vi "Global Variable.vi"() -> ()   [LabVIEW 2018]
panel:
  out "PicoScope Device Info":T1
  out "BLE Data":string
  out "PicoScope Correction":i32
  out "FTDI RS232 Handle  RFID":u32
  out "Baccode MEM":string
  in  "VI Refnum Main":refnum<vi>
  out "Steps Cnt":u16
  out "Sequencer Path":path[](array[path])=[path "***", path "***", path "***", path "***", path "***", path "***", path "***", path "***", path "***", path "***"]
  out "logFile Path":refnum<file>
  out "Reset BARCODE":bool
  out "Retest Nmb":i16
  out "Boards False":u32
  out "Boards Pass":u32
  out "Boards Total":u32
  out "DB Dir Path":path caption="Sequenser INI Config File Path"
  out "Config":string="***"
  out "Board":string="***"
  out "Customer":string="***"
  out "Gen Err Cnt":u16
  out "Cancel by operator":bool
  out "RFID Power":u16
  out "Retest Step Nmb":u32
  out "Retest ON":bool
  out "Retest Cnt":i16
  out "Rd PID RFID":string
  out "COM Port RFID":refnum<visa-resource-name>
  in  "VI Ref PicoScope Read":refnum<vi>
  out "Test Gen Status":bool
  out "COM Port BLE":refnum<visa-resource-name>
  out "Rd PID Ble":string
  out "ADC Offset":i32
  out "Test Time":u32
  out "Test Stop Time":u32
  out "Test Start Time":u32
  out "Array_Measurement":dbl[](array[numeric]) format="%#.3g"
  out "Rd PID":string
  out "Wr PID":string
  out "COM Port FTDI RS232":refnum<visa-resource-name>
  out "PowSupply ON/OFF":bool
  out "GPIO Mode LUT":bool[](array[boolean])
  out "PicoScope Max Adc Value":i16
  out "PicoScope Handle":u32
  in  "Step Test Result":enum16{"Idle", "PASS", "FALSE"}(ring)
  out "Report Active Lines Cnt":u32
  out "Report Step Nmb":u32
  out "Active Lines Cnt":u32
  out "VISA Resource Name BK-5492C":string
  out "VISA Resource Name BK-9202":string
  out "Simbol Array":u32[](array[numeric])
  out "Current Step Nmb":u32
  out "Steps Nmb":u32
  out "FTDI RS232 Handle":u32
  out "FTDI SPI Handle":u32
  out "Array Errors":errorcluster[](array[cluster])
  out "Sys ERR":bool
  out "Dev List":string[](array[string])
  out "System Status":T2(ring)
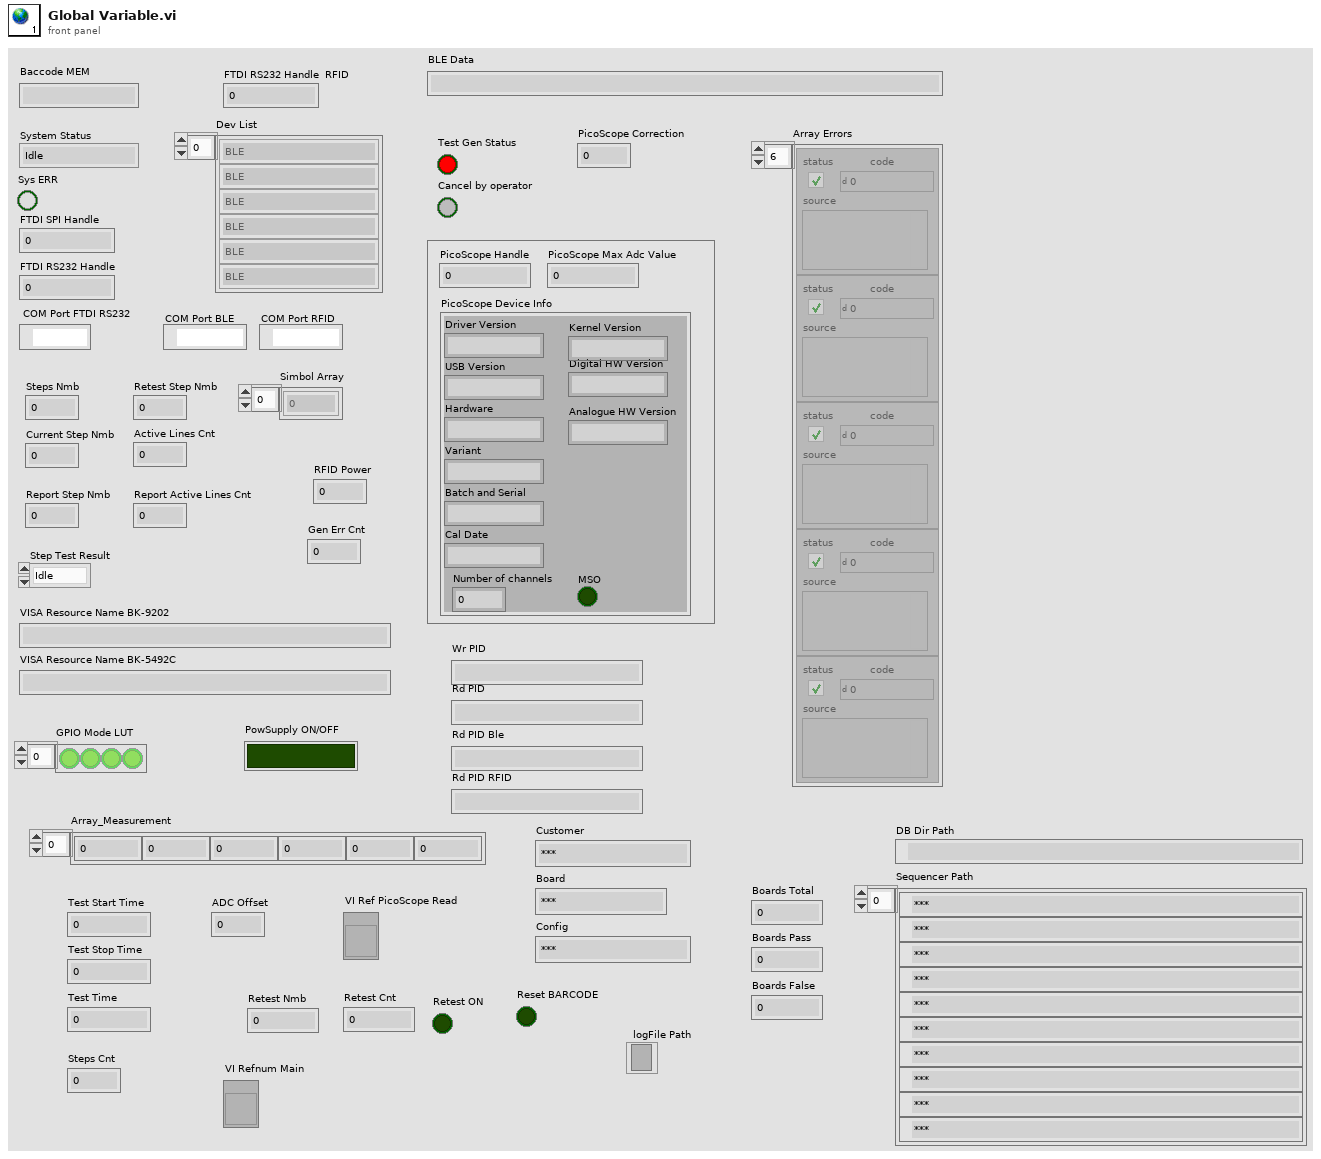
[diagram p1: front panel]
types:
  T1 = cluster{"Driver Version":string, "USB Version":string, "Hardware":string, "Variant":string, "Batch and Serial":string, "Cal Date":string, "Kernel Version":string, "Digital HW Version":string, "Analogue HW Version":string, "MSO":bool, "Number of channels":i16}
  T2 = enum16{"Idle", "INI System", "INI Devices", "START Sequencer", "INI Secuencer", "Run Sequencer", "STOP Sequencer", "Report Generation", "Test Load Monitor", "QUIT"}
diagram:
